vi "Log GoTo State Helper.vi"(7 "State Info":string, 8 "error in (no error)":errorcluster, 9 "GoTo Cmd":T1, 10 "Data":i32, 11 "EventLog in":refnum<class "EventLog.lvclass">) -> (0 "error out":errorcluster, 3 "EventLog out":refnum<class "EventLog.lvclass">)   [LabVIEW 2015, in "Tool Module.lvlib"]
uses:
  Tool Module.lvlib
  QC-X App/Libraries/Event Logger Library/Event Log/EventLog.lvclass
  _GoTo Cmd Typedef--enum.ctl
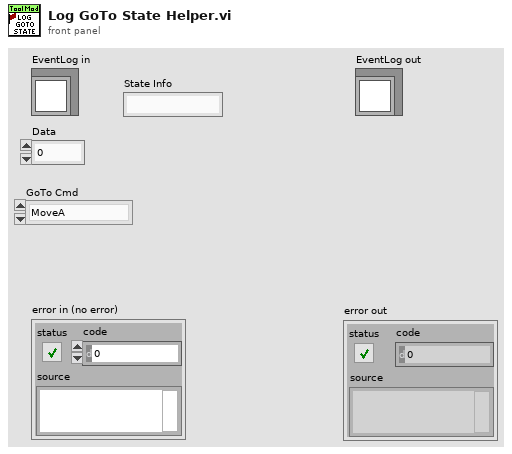
[diagram p1: front panel]
types:
  T1 = typedef "Tool Module.lvlib/_GoTo Cmd Typedef--enum.ctl" = enum16{"MoveA", "MoveR", "Home Position", "Home None", "Cleaning Position"}
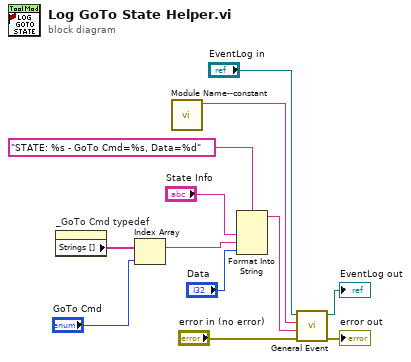
[diagram p0: block diagram]
diagram:
  n1 = property on="_GoTo Cmd typedef" class="Enum (strict)"() -> ("Strings []"=w3:string[])  [unwired: 2 in, 2 out]
  n2 = Index Array(array=w3, index="GoTo Cmd") -> (element=w2:string)
  n3 = call "Module Name--constant.vi"() -> ("Module Name"=w4:string)  [unwired: 11 in]
  n4 = Format Into String(format string="STATE: %s - GoTo Cmd=%s, Data=%d", "State Info", w2, "Data") -> (resulting string=w12:string)  [unwired: 2 in, 1 out]
  n5 = call "General Event.vi"("error in (no error)"="error in (no error)", "Event Description"=w12, "Event Name"=w4, "EventLog ref"="EventLog in") -> ("error out"=→"error out":errorcluster, "EventLog ref"=→"EventLog out":refnum<class "EventLog.lvclass">)  [unwired: 6 in]
